vi "Create Parameterized Executive.vi"(4 "File Name":string, 6 "Folder":path, 7 "Attribute Name Blacklist":string[](array[string]), 8 "error in (no error)":errorcluster, 9 "Persistence in":refnum<class "IPersist.lvclass">, 10 "Test Executive":refnum<class "ITest Executive.lvclass">, 11 "ITest Executive in":refnum<class "ITest Executive.lvclass">) -> (0 "error out":errorcluster, 3 "ITest Executive out":refnum<class "ITest Executive.lvclass">)   [LabVIEW 2019, in "Test Executive.lvlib" / "ITest Executive.lvclass"]
uses:
  <vilib>/gpm_packages/@cs/test-executive/Source/Test Executive/ITestExecutive/ITest Executive.lvclass
  <vilib>/gpm_packages/@cs/persistence/source/IPersist/IPersist.lvclass
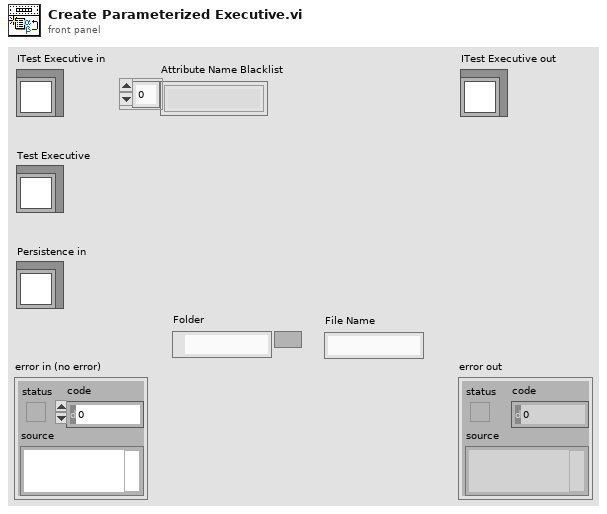
[diagram p1: front panel]
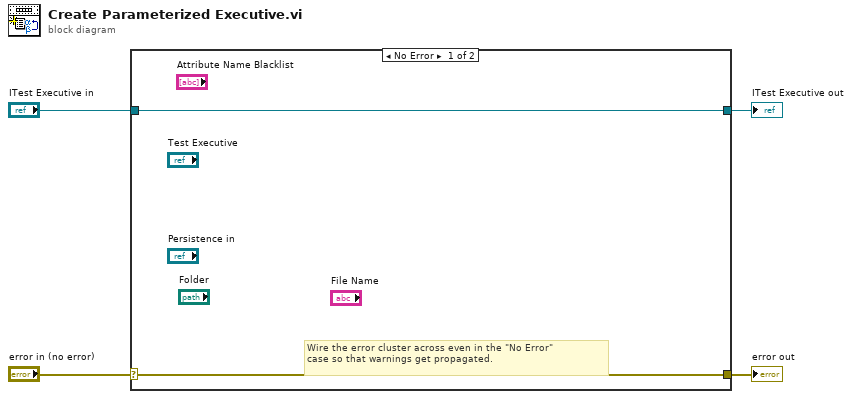
[diagram p0: block diagram]
diagram:
  n1 = case shown="No Error" "error in (no error)" {
    selector: "error in (no error)" -> [w5 w8]
    tunnel: [w5 w8] -> w3
    tunnel: [w6 w7] -> w1
    tunnel: "ITest Executive in" -> [w6 w7]
    frame No Error {
      # "Wire the error cluster across even in the \"No Error\"\ncase so that warnings get propagated."
    }
    frame Error {
    }
  }
  "error out" <- w3
  "ITest Executive out" <- w1
